vi "GUNSC_API.vi"(0 "modpath":path, 7 "Cmd":string, 11 "error in":errorcluster) -> (4 "ImmedReplyString":string, 15 "error out":errorcluster)   [LabVIEW 2014]
uses:
  DBSHAND/private/vis/DatabaseHand_Element_Set(string).vi
  DBSHAND/private/vis/DatabaseHand_Element_Set(bool).vi
panel:
  out "caller path":path
  in  "Module vi name":string="GUNSC_Main.vi"
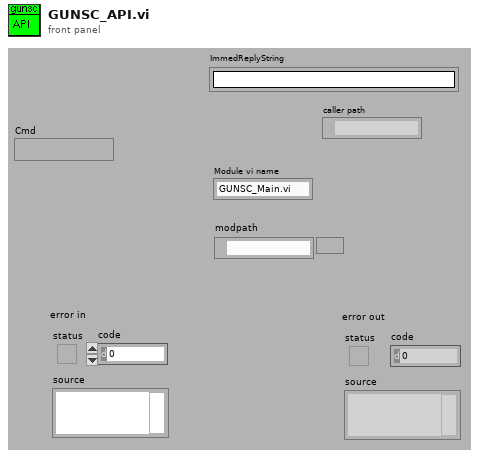
[diagram p1: front panel]
types:
  T1 = typedef "DatabaseHand_RefNum.ctl" = refnum<vi>
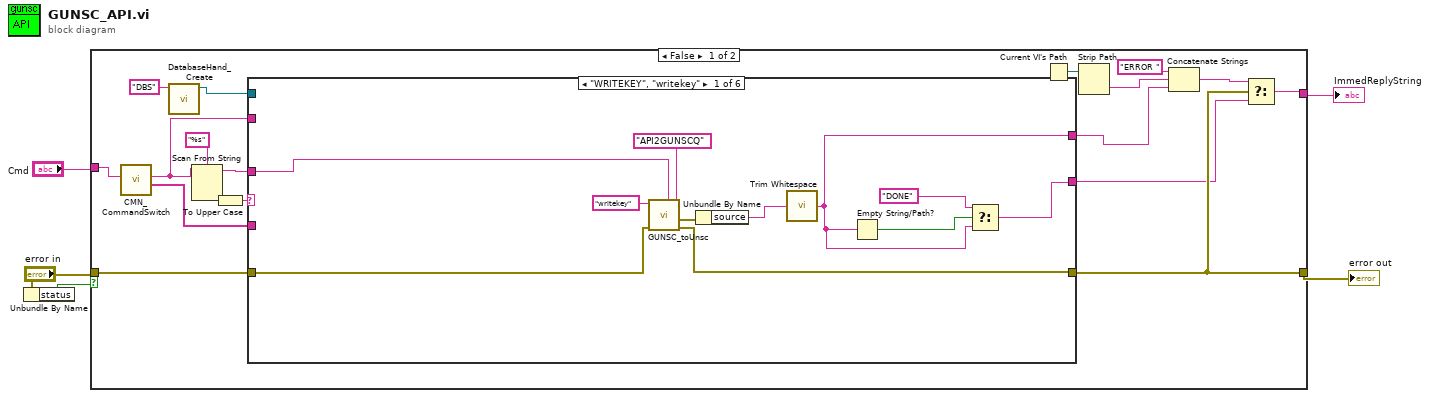
[diagram p0: block diagram]
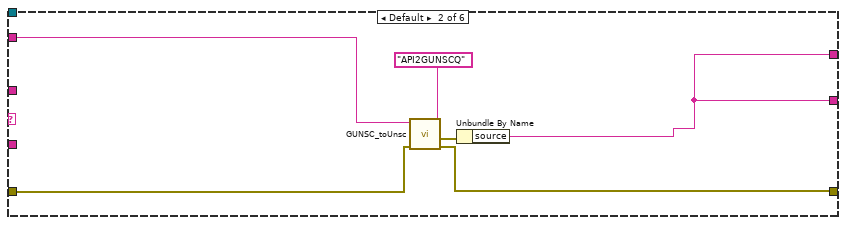
[diagram p2: hidden frame]
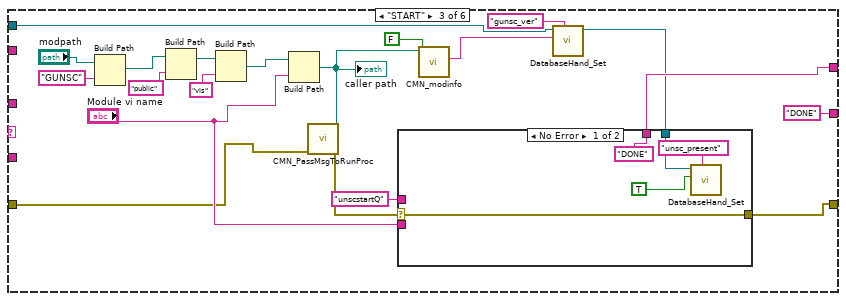
[diagram p3: hidden frame]
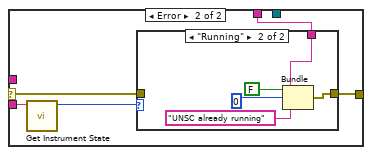
[diagram p4: hidden frame]
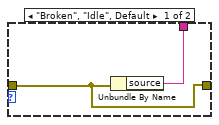
[diagram p5: hidden frame]
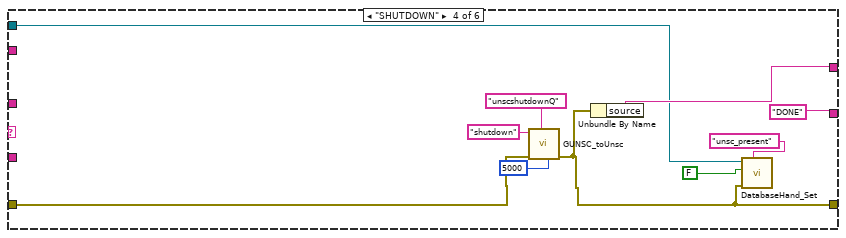
[diagram p6: hidden frame]
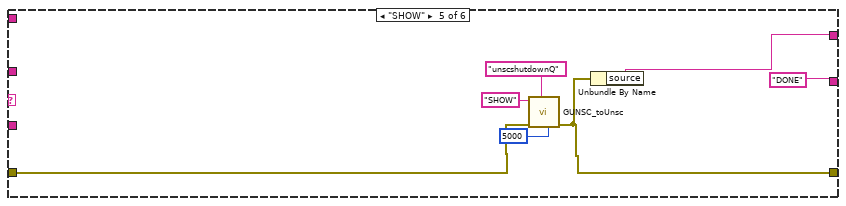
[diagram p7: hidden frame]
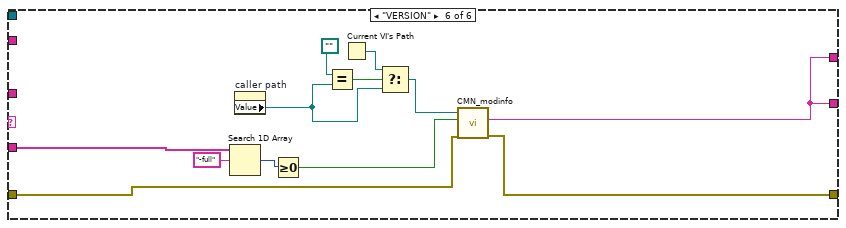
[diagram p8: hidden frame]
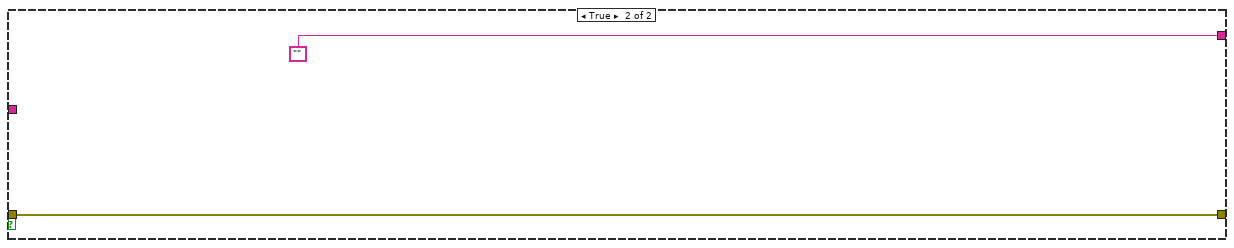
[diagram p9: hidden frame]
diagram:
  n1 = Unbundle By Name("error in") -> ("status"=w3:bool)
  n2 = case shown="False" w3 {
    tunnel: "error in" -> [w23 w107]
    tunnel: [w16 w107] -> w1
    tunnel: [w15 ""] -> w5
    tunnel: "Cmd" -> [w12 _]
    frame False {
      n3 = call "CMN_CommandSwitch.vi"("command in"=w12) -> ("swhitches"=w11:string[], "command out"=w8:string)  [unwired: 1 in, 8 out]
      n4 = call "DatabaseHand_Create.vi"("Name"="DBS") -> ("Database RefNum out"=w6:T1)  [unwired: 1 in, 9 out]
      n5 = Scan From String(format string="%s" ("Format String"), input string=w8) -> (remaining string=w10:string, output 1=w22:string)  [unwired: 2 in, 3 out]
      n6 = To Upper Case(1:w22) -> (0:w9:string)
      n7 = case shown="\"WRITEKEY\", \"writekey\"" w9 {
        tunnel: w23 -> [w32 w40 w43 w85 w92 w101]
        tunnel: [w31 w39 w59 w79 w91 w100] -> w16
        tunnel: [w24 w35 w45 w84 w90 w99] -> w14
        tunnel: [w25 w35 "DONE" "DONE" "DONE" w99] -> w13
        tunnel: w11 -> [_ _ _ _ _ w102]
        tunnel: w10 -> [w33 _ _ _ _ _]
        tunnel: w8 -> [_ w36 _ _ _ _]
        tunnel: w6 -> [_ _ w41 w78 _ _]
        frame "WRITEKEY", "writekey" {
          n8 = call "GUNSC_toUnsc.vi"("responseQ"="API2GUNSCQ", "key"=w33, "error in (no error)"=w32, "command"="writekey") -> ("error out"=w31:errorcluster, "response"=w29:errorcluster)  [unwired: 5 in, 1 out]
          n9 = Unbundle By Name(w29) -> ("source"=w28:string)
          n10 = call <vilib>:"Trim Whitespace.vi"("string"=w28) -> ("trimmed string"=w24:string)  [unwired: 1 in]
          n11 = Empty String/Path?(string/path=w24) -> (empty?=w27:bool)
          n12 = Select(t="DONE" ("INFO"), s=w27, f=w24) -> (s? t:f=w25:string)
        }
        frame Default {
          n13 = call "GUNSC_toUnsc.vi"("responseQ"="API2GUNSCQ", "error in (no error)"=w40, "command"=w36) -> ("error out"=w39:errorcluster, "response"=w37:errorcluster)  [unwired: 6 in, 1 out]
          n14 = Unbundle By Name(w37) -> ("source"=w35:string)
        }
        frame "START" {
          n15 = Build Path(base path="modpath", name or relative path="GUNSC") -> (appended path=w54:path)
          n16 = Build Path(base path=w54, name or relative path="public") -> (appended path=w52:path)
          n17 = Build Path(base path=w52, name or relative path="vis") -> (appended path=w50:path)
          n18 = Build Path(base path=w50, name or relative path="Module vi name") -> (appended path=w44:path)
          "caller path" <- w44
          n19 = call "CMN_PassMsgToRunProc.vi"("VItoRun"=w44, "error in (no error)"=w43) -> ("error out"=w60:errorcluster)  [unwired: 1 in, 12 out]
          n20 = call "CMN_modinfo.vi"("full"=FALSE, "caller path"=w44) -> ("INFO"=w46:string)  [unwired: 1 in, 8 out]
          n21 = call-poly "DatabaseHand_Set.vi"("name"="gunsc_ver", "value"=w46, "Database RefNum in"=w41) -> ("Database RefNum out"=w42:T1)  [unwired: 5 in, 3 out]
          n22 = case shown="No Error" w60 {
            selector: w60 -> [w65 w69]
            tunnel: [w65 w66] -> w59
            tunnel: ["DONE" ("source") w67] -> w45
            tunnel: "unscstartQ" ("name (unnamed)") -> [_ _]
            tunnel: "Module vi name" -> [_ w68]
            tunnel: w42 -> [w63 _]
            frame No Error {
              n23 = call-poly "DatabaseHand_Set.vi"("name"="unsc_present", "value"=TRUE ("full"), "Database RefNum in"=w63) -> ()  [unwired: 5 in, 4 out]
            }
            frame Error {
              n24 = call <vilib>:"Get Instrument State.vi"("VI name"=w68) -> ("vi state"=w70:enum32{"Broken", "Idle", "Running"})  [unwired: 1 in, 9 out]
              n25 = case shown="\"Running\"" w70 {
                tunnel: w69 -> [w71 _]
                tunnel: [w72 w73] -> w67
                tunnel: [w71 w76] -> w66
                frame "Broken", "Idle", Default {
                  n26 = Unbundle By Name(w71) -> ("source"=w72:string)
                }
                frame "Running" {
                  w73 = "UNSC already running"
                  n27 = Bundle(FALSE, 0, w73) -> (w76:errorcluster)  [unwired: 1 out]
                }
              }
            }
          }
        }
        frame "SHUTDOWN" {
          n28 = call "GUNSC_toUnsc.vi"("responseQ"="unscshutdownQ", "ms timeout (-1)"=5000, "error in (no error)"=w85, "command"="shutdown" ("Command")) -> ("error out"=w79:errorcluster)  [unwired: 5 in, 2 out]
          n29 = Unbundle By Name(w79) -> ("source"=w84:string)
          n30 = call-poly "DatabaseHand_Set.vi"("name"="unsc_present", "error in (no error)"=w79, "value"=FALSE ("full"), "Database RefNum in"=w78) -> ()  [unwired: 4 in, 4 out]
        }
        frame "SHOW" {
          n31 = call "GUNSC_toUnsc.vi"("responseQ"="unscshutdownQ", "ms timeout (-1)"=5000, "error in (no error)"=w92, "command"="SHOW" ("Command")) -> ("error out"=w91:errorcluster)  [unwired: 5 in, 2 out]
          n32 = Unbundle By Name(w91) -> ("source"=w90:string)
        }
        frame "VERSION" {
          n33 = Search 1D Array(1D array=w102, element="-full") -> (index of element=w104:i32)  [unwired: 1 out]
          n34 = property on="caller path" class="Path"() -> ("Value"=w95:path)  [unwired: 2 in, 2 out]
          n35 = Greater Or Equal To 0?(x=w104) -> (x >= 0?=w103:bool)
          n36 = Equal?(x=path "", y=w95) -> (x = y?=w97:bool)
          n37 = Current VI's Path() -> (path=w96:path)
          n38 = Select(t=w96, s=w97, f=w95) -> (s? t:f=w94:path)
          n39 = call "CMN_modinfo.vi"("error in (no error)"=w101, "full"=w103, "caller path"=w94) -> ("error out"=w100:errorcluster, "INFO"=w99:string)  [unwired: 7 out]
        }
      }
      n40 = Current VI's Path() -> (path=w19:path)
      n41 = Strip Path(path=w19) -> (name=w18:string)  [unwired: 1 out]
      n42 = Concatenate Strings("ERROR ", w18, w14) -> (w17:string)
      n43 = Select(t=w17, s=w16, f=w13) -> (s? t:f=w15:string)
    }
    frame True {
    }
  }
  "error out" <- w1
  "ImmedReplyString" <- w5
